vi "WPI_CameraGet Brightness.vi"(8 "error in (no error)":errorcluster, 11 "CameraDevRef":T1={"Camera Address"="192.168.0.90", "CameraStatus"={"status"=FALSE, "code"=0, "source"=""}}) -> (0 "error out":errorcluster, 2 "Brightness":i32, 3 "CameraDevRef Out":T1)   [LabVIEW 2017]
doc: "Returns the brightness setting of the camera you specify.\n\nThis software is licensed. Open the labview\\readme\\WPI Robotics Library Open Source License.txt file for more information."
uses:
  <vilib>/Rock Robotics/WPI/Camera/WPI_CameraDevRef.ctl
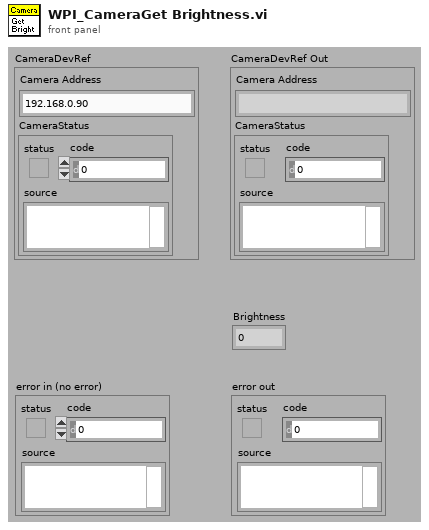
[diagram p1: front panel]
types:
  T1 = typedef "WPI_CameraDevRef.ctl" = cluster{"Camera Address":string, "CameraStatus":errorcluster}
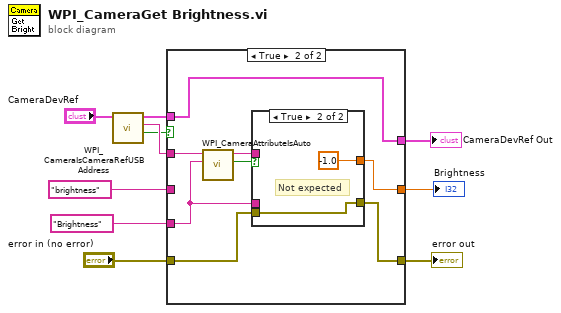
[diagram p0: block diagram]
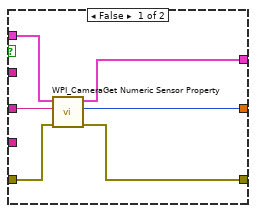
[diagram p2: hidden frame]
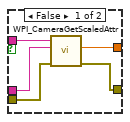
[diagram p3: hidden frame]
diagram:
  n1 = call <vilib>:"WPI_CameraIsCameraRefUSBAddress.vi"("CameraDevRef"="CameraDevRef") -> ("USB?"=w1:bool, "Camera Address Out"=w2:string, "CameraDevRef out"=w3:T1)  [unwired: 7 in, 1 out]
  n2 = case shown="True" w1 {
    tunnel: [w16 w19] -> w10
    tunnel: "brightness" ("Property Name") -> [w15 _]
    tunnel: [w14 w20] -> w8
    tunnel: "error in (no error)" -> [w13 w18]
    tunnel: [w12 w17] -> w6
    tunnel: w3 -> [w11 w19]
    tunnel: w2 -> [_ w22]
    tunnel: "Brightness" ("Property Name") -> [_ w21]
    frame False {
      n3 = call <vilib>:"WPI_CameraGet Numeric Sensor Property.vi"("error in (no error)"=w13, "Property Name"=w15, "CameraDevRef"=w11) -> ("error out"=w12:errorcluster, "Value"=w14:i32, "CameraDevRef dup"=w16:T1)  [unwired: 2 in, 4 out]
    }
    frame True {
      n4 = call <vilib>:"WPI_CameraAttributeIsAuto.vi"("Attr String"=w21, "Camera Address In"=w22) -> ("Auto?"=w24:bool, "Camera Address Out"=w23:string)  [unwired: 8 in]
      n5 = case shown="True" w24 {
        tunnel: w21 -> [w28 _]
        tunnel: w23 -> [w29 _]
        tunnel: [w27 -1.0] -> w20
        tunnel: w18 -> [w26 w30]
        tunnel: [w25 w30] -> w17
        frame False {
          n6 = call <vilib>:"WPI_CameraGetScaledAttr.vi"("error in (no error)"=w26, "Attr String"=w28, "Camera Address In"=w29) -> ("error out"=w25:errorcluster, "Scaled"=w27:dbl)  [unwired: 5 in, 2 out]
        }
        frame True {
          # "Not expected"
        }
      }
    }
  }
  "CameraDevRef Out" <- w10
  "Brightness" <- w8
  "error out" <- w6
